vi "Init Test Result Data.vi"(8 "error in (no error)":errorcluster, 10 "Result.lvclass":refnum<class "Test Result.lvclass">, 11 "Test Step in":refnum<class "Test Step.lvclass">) -> (0 "error out":errorcluster, 3 "Test Step out":refnum<class "Test Step.lvclass">)   [LabVIEW 2021, in "Sequence Engine.lvlib" / "Test Step.lvclass"]
uses:
  Test Step.lvclass
  Test Result/Test Result.lvclass
  Test Step.lvclass/Test Step.ctl
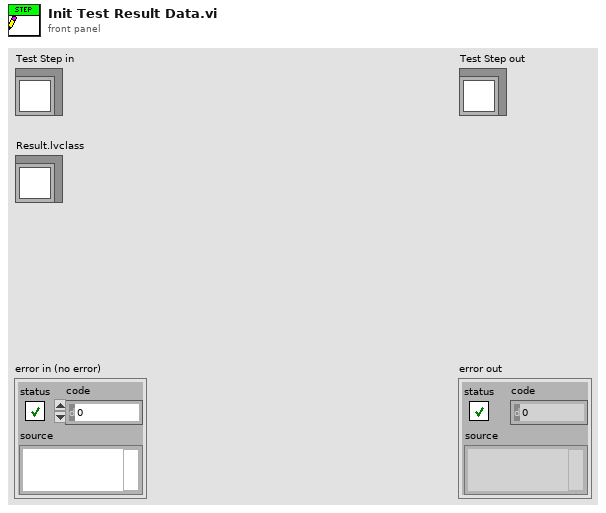
[diagram p1: front panel]
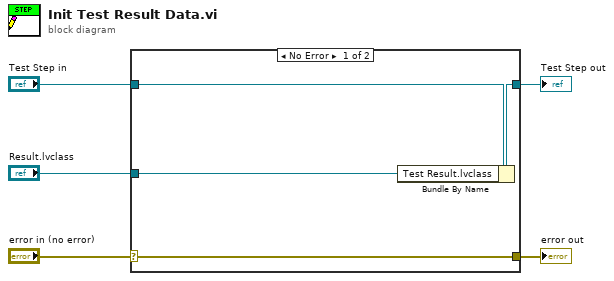
[diagram p0: block diagram]
diagram:
  n1 = case shown="No Error" "error in (no error)" {
    selector: "error in (no error)" -> [w9 w10]
    tunnel: [w9 w10] -> w4
    tunnel: [w7 w11] -> w2
    tunnel: "Test Step in" -> [w8 w11]
    tunnel: "Result.lvclass" -> [w6 _]
    frame No Error {
      n2 = Bundle By Name(cluster=w8, "Test Result.lvclass"=w6) -> (w7:refnum<class "Test Step.lvclass">)
    }
    frame Error {
    }
  }
  "error out" <- w4
  "Test Step out" <- w2
